vi "threshold for 2nd mom.vi"(8 "error in (no error)":errorcluster, 9 "mask":T1, 10 "Image Dst Out":T1, 11 "Refnum in":T1) -> (0 "error out":errorcluster, 3 "Refnum out":T1)   [LabVIEW 2020, in "Point Grey Camera.lvclass"]
uses:
  Point Grey Camera.lvclass
  IMAQ Image.ctl
  NI_Vision_Development_Module.lvlib
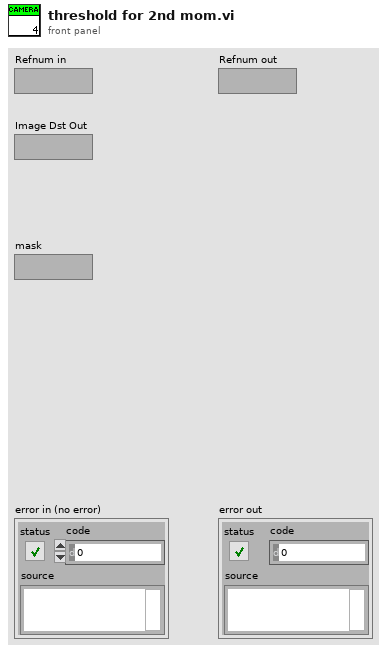
[diagram p1: front panel]
types:
  T1 = typedef "IMAQ Image.ctl" = refnum<image>
  T2 = cluster{"histogram":u32[], "Minimal Value":sgl, "Maximal Value":sgl, "Starting Value":sgl, "Interval Width":sgl, "Mean Value":sgl, "Standard  Variation":sgl, "Area (pixels)":i32}
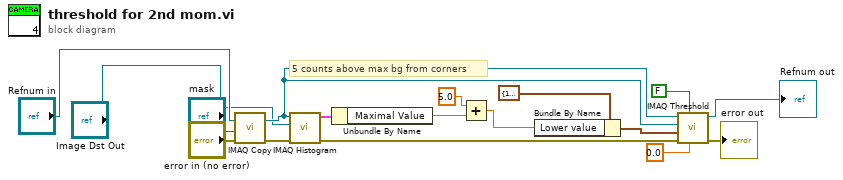
[diagram p0: block diagram]
diagram:
  # "5 counts above max bg from corners"
  n1 = call "IMAQ Copy"("error in (no error)"="error in (no error)", "Image Dst"="Image Dst Out", "Image Src"="Refnum in") -> ("error out"=w16:errorcluster, "Image Dst Out"=w12:T1)  [unwired: 3 in]
  n2 = call "IMAQ Histogram"("error in (no error)"=w16, "Image Mask"="mask", "Image"=w12) -> ("error out"=w11:errorcluster, "Histogram Report"=w4:T2)  [unwired: 7 in]
  n3 = Unbundle By Name(w4) -> ("Maximal Value"=w3:sgl)
  n4 = Add(x=sgl 5.0, y=w3) -> (x+y=w2:sgl)
  n5 = Bundle By Name(cluster=cluster{"Lower value":sgl, "Upper value":sgl} {"Lower value"=100.0, "Upper value"=9999999.0} ("Range"), "Lower value"=w2) -> (w6:cluster{"Lower value":sgl, "Upper value":sgl})
  n6 = call "IMAQ Threshold"("Replace Value"=sgl 0.0, "Keep/Replace Value (Replace)"=FALSE, "error in (no error)"=w11, "Range"=w6, "Image Dst"=w12, "Image Src"=w12) -> ("error out"=→"error out":errorcluster, "Image Dst Out"=→"Refnum out":T1)  [unwired: 4 in]
